vi "start.vi"(8 "error in (no error)":errorcluster, 11 "EncoderConverter in":refnum<class "EncoderConverter.lvclass">) -> (0 "error out":errorcluster, 3 "EncoderConverter out":refnum<class "EncoderConverter.lvclass">)   [LabVIEW 2013, in "EncoderConverter.lvlib" / "EncoderConverter.lvclass"]
uses:
  <userlib>/Common/Devices/EncoderConverter/EncoderConverter/EncoderConverter.lvclass
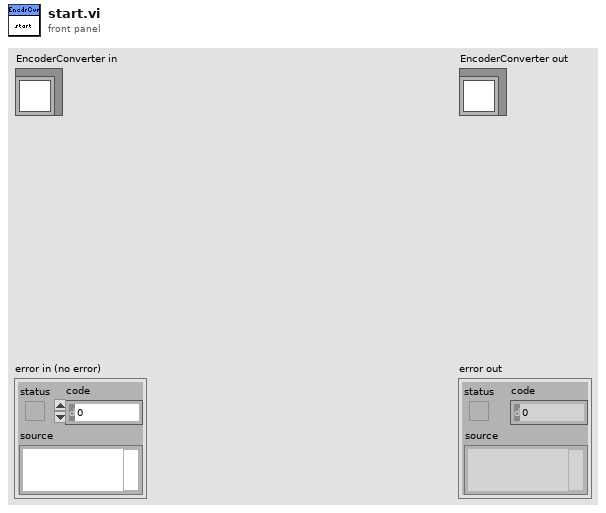
[diagram p1: front panel]
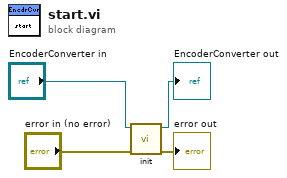
[diagram p0: block diagram]
diagram:
  n1 = call <userlib>:"init.vi"("error in (no error)"="error in (no error)", "Encoder in"="EncoderConverter in") -> ("error out"=→"error out":errorcluster, "Encoder out"=→"EncoderConverter out":refnum<class "EncoderConverter.lvclass">)  [unwired: 8 in]
